vi "StateAlarmManagement.vi"(0 "Master State In":T1(ring)) -> ()   [LabVIEW 2020]
doc: "This VI manages the Master ALARM and master CAUTION states for the robot."
uses:
  GlobalPoseAndTargeting.vi
  GlobalDriverStationData.vi
  GlobalAutonomous.vi
  GlobalDrivebase.vi
  GlobalMiscellaneous.vi
  GlobalArm.vi
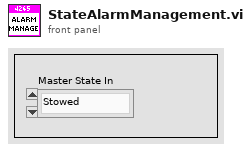
[diagram p1: front panel]
types:
  T1 = enum16{"Stowed", "Balancing", "Scoring", "Hoppering", "Ground", "Shelf"}
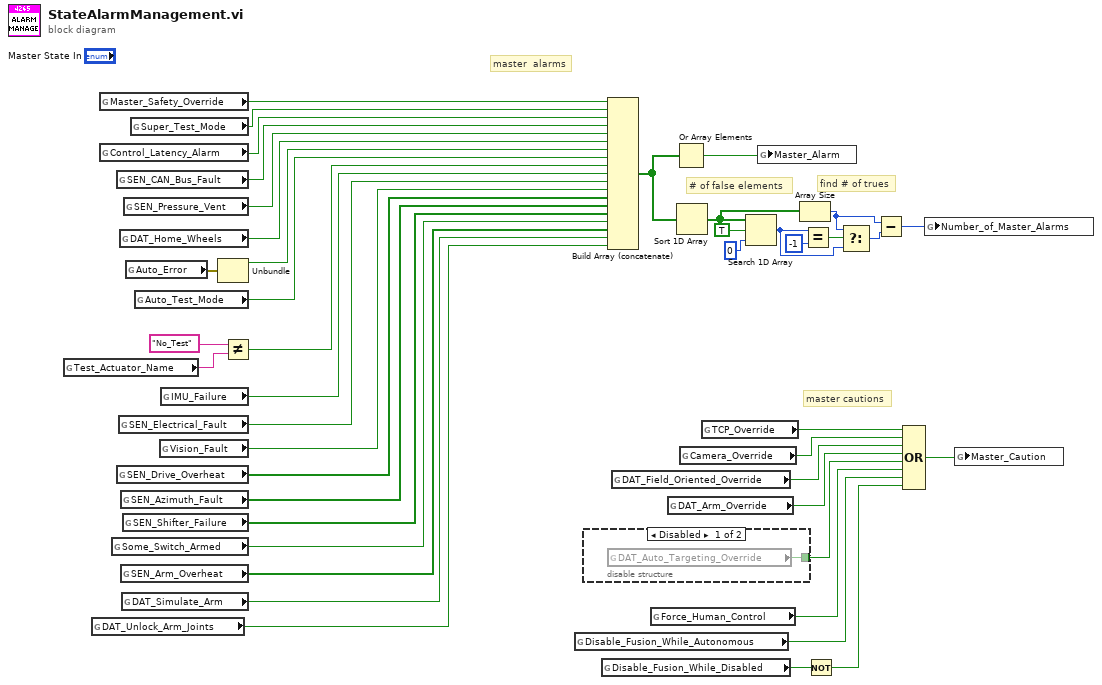
[diagram p0: block diagram]
diagram:
  # "master cautions"
  # "master  alarms"
  # "# of false elements"
  # "find # of trues"
  n1 = global read "GlobalDriverStationData.vi" "Test_Actuator_Name"() -> (w37:string)
  n2 = global read "GlobalArm.vi" "DAT_Unlock_Arm_Joints"() -> (w1:bool)
  n3 = global read "GlobalDriverStationData.vi" "Master_Safety_Override"() -> (w43:bool)
  n4 = global read "GlobalMiscellaneous.vi" "Control_Latency_Alarm"() -> (w18:bool)
  n5 = global read "GlobalDriverStationData.vi" "Some_Switch_Armed"() -> (w12:bool)
  n6 = global read "GlobalMiscellaneous.vi" "SEN_CAN_Bus_Fault"() -> (w17:bool)
  n7 = global read "GlobalDrivebase.vi" "SEN_Drive_Overheat"() -> (w15:bool[])
  n8 = global read "GlobalMiscellaneous.vi" "SEN_Electrical_Fault"() -> (w19:bool)
  n9 = global read "GlobalDrivebase.vi" "DAT_Home_Wheels"() -> (w20:bool)
  n10 = global read "GlobalDrivebase.vi" "SEN_Azimuth_Fault"() -> (w14:bool[])
  n11 = global read "GlobalArm.vi" "SEN_Arm_Overheat"() -> (w11:bool[])
  n12 = global read "GlobalArm.vi" "DAT_Simulate_Arm"() -> (w10:bool)
  n13 = global read "GlobalDrivebase.vi" "SEN_Shifter_Failure"() -> (w13:bool[])
  n14 = global read "GlobalMiscellaneous.vi" "SEN_Pressure_Vent"() -> (w16:bool)
  n15 = global read "GlobalAutonomous.vi" "Auto_Error"() -> (w41:errorcluster)
  n16 = global read "GlobalDriverStationData.vi" "Super_Test_Mode"() -> (w42:bool)
  n17 = global read "GlobalDriverStationData.vi" "Auto_Test_Mode"() -> (w39:bool)
  n18 = global read "GlobalPoseAndTargeting.vi" "Vision_Fault"() -> (w34:bool)
  n19 = global read "GlobalPoseAndTargeting.vi" "IMU_Failure"() -> (w35:bool)
  n20 = Unbundle(w41) -> ("status"=w40:bool)  [unwired: 2 out]
  n21 = Not Equal?(x="No_Test", y=w37) -> (x != y?=w36:bool)
  n22 = global read "GlobalDriverStationData.vi" "Disable_Fusion_While_Autonomous"() -> (w4:bool)
  n23 = disable-structure shown="Disabled" {
    disable-tunnel: [w44 _] -> w6
    frame Disabled {
      n24 = global read "GlobalDrivebase.vi" "DAT_Auto_Targeting_Override"() -> (w44:bool)
    }
    frame Enabled {
    }
  }
  n25 = global read "GlobalDriverStationData.vi" "Disable_Fusion_While_Disabled"() -> (w3:bool)
  n26 = Build Array (concatenate)(w43, w42, w18, w17, w16, w20, w40, w39, w36, w35, w19, w34, w15, w14, w13, w12, w11, w10, w1) -> (w25:bool[])
  n27 = global read "GlobalDrivebase.vi" "DAT_Field_Oriented_Override"() -> (w8:bool)
  n28 = global read "GlobalDriverStationData.vi" "Force_Human_Control"() -> (w5:bool)
  n29 = global read "GlobalArm.vi" "DAT_Arm_Override"() -> (w7:bool)
  n30 = Or Array Elements(Boolean array=w25) -> (logical OR=w24:bool)
  n31 = Sort 1D Array(array=w25) -> (sorted array=w30:bool[])
  n32 = global read "GlobalDriverStationData.vi" "Camera_Override"() -> (w9:bool)
  n33 = global read "GlobalDriverStationData.vi" "TCP_Override"() -> (w22:bool)
  n34 = Search 1D Array(1D array=w30, element=TRUE, start index (0)=0) -> (index of element=w33:i32)
  n35 = global write "GlobalMiscellaneous.vi" "Master_Alarm"(w24) -> ()
  n36 = Array Size(array=w30) -> (size(s)=w32:i32)
  n37 = Equal?(x=w33, y=-1) -> (x = y?=w29:bool)
  n38 = Not(x=w3) -> (.not. x?=w2:bool)
  n39 = Select(t=w32, s=w29, f=w33) -> (s? t:f=w31:i32)
  n40 = Subtract(x=w32, y=w31) -> (x-y=w23:i32)
  n41 = Compound Arithmetic op=OR(w22, w9, w8, w7, w6, w5, w4, w2) -> (w21:bool)
  n42 = global write "GlobalMiscellaneous.vi" "Number_of_Master_Alarms"(w23) -> ()
  n43 = global write "GlobalMiscellaneous.vi" "Master_Caution"(w21) -> ()
